vi "range_inc.vi"(8 "Error In":errorcluster, 10 "Unit":string, 11 "Amp":dbl) -> (0 "Error Out":errorcluster, 2 "Amp Base":dbl, 3 "Amp String":dbl)   [LabVIEW 2021, in "Signal.lvlib"]
doc: "This VI is used to check the range while incrementing or decrementing."
uses:
  Signal.lvlib
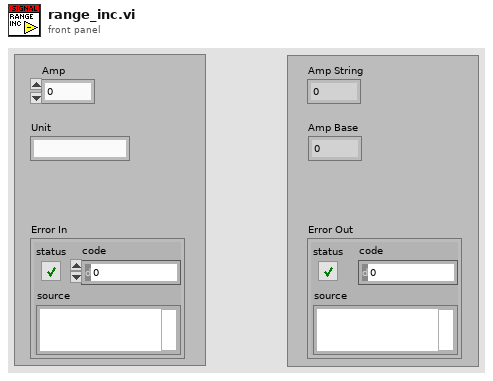
[diagram p1: front panel]
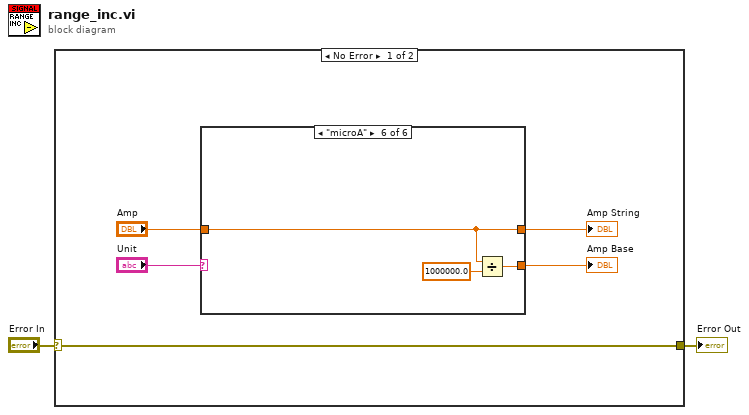
[diagram p0: block diagram]
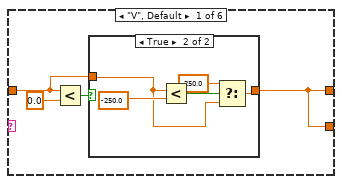
[diagram p2: hidden frame]
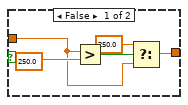
[diagram p3: hidden frame]
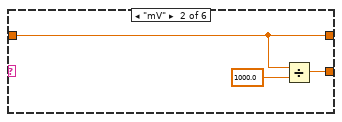
[diagram p4: hidden frame]
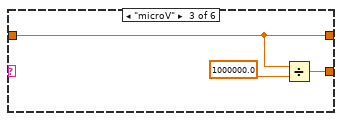
[diagram p5: hidden frame]
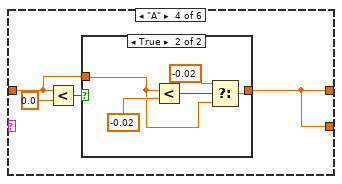
[diagram p6: hidden frame]
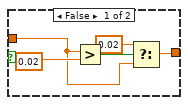
[diagram p7: hidden frame]
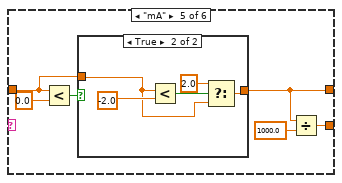
[diagram p8: hidden frame]
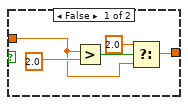
[diagram p9: hidden frame]
diagram:
  n1 = case shown="No Error" "Error In" {
    selector: "Error In" -> [w3 w61]
    tunnel: [w3 w61] -> w1
    frame No Error {
      n2 = case shown="\"microA\"" "Unit" {
        tunnel: "Amp" -> [w8 w23 w26 w29 w45 w59]
        tunnel: [w11 w22 w25 w28 w43 w60] -> w6
        tunnel: [w11 w23 w26 w28 w44 w59] -> w7
        frame "V", Default {
          n3 = Less?(x=w8, y=0.0) -> (x < y?=w9:bool)
          n4 = case shown="True" w9 {
            tunnel: [w13 w17] -> w11
            tunnel: w8 -> [w12 w18]
            frame False {
              n5 = Greater?(x=w12, y=250.0) -> (0:w15:bool)
              n6 = Select(t=250.0, s=w15, f=w12) -> (s? t:f=w13:dbl)
            }
            frame True {
              n7 = Less?(x=w18, y=-250.0) -> (x < y?=w20:bool)
              n8 = Select(t=-250.0, s=w20, f=w18) -> (s? t:f=w17:dbl)
            }
          }
        }
        frame "mV" {
          n9 = Divide(x=w23, y=1000.0) -> (x/y=w22:dbl)
        }
        frame "microV" {
          n10 = Divide(x=w26, y=1000000.0) -> (x/y=w25:dbl)
        }
        frame "A" {
          n11 = Less?(x=w29, y=0.0) -> (x < y?=w30:bool)
          n12 = case shown="True" w30 {
            tunnel: [w33 w37] -> w28
            tunnel: w29 -> [w32 w38]
            frame False {
              n13 = Greater?(x=w32, y=0.02) -> (0:w35:bool)
              n14 = Select(t=0.02, s=w35, f=w32) -> (s? t:f=w33:dbl)
            }
            frame True {
              n15 = Less?(x=w38, y=-0.02) -> (x < y?=w40:bool)
              n16 = Select(t=-0.02, s=w40, f=w38) -> (s? t:f=w37:dbl)
            }
          }
        }
        frame "mA" {
          n17 = Less?(x=w45, y=0.0) -> (x < y?=w46:bool)
          n18 = case shown="True" w46 {
            tunnel: [w49 w53] -> w44
            tunnel: w45 -> [w48 w54]
            frame False {
              n19 = Greater?(x=w48, y=2.0) -> (0:w51:bool)
              n20 = Select(t=2.0, s=w51, f=w48) -> (s? t:f=w49:dbl)
            }
            frame True {
              n21 = Less?(x=w54, y=-2.0) -> (x < y?=w56:bool)
              n22 = Select(t=2.0, s=w56, f=w54) -> (s? t:f=w53:dbl)
            }
          }
          n23 = Divide(x=w44, y=1000.0) -> (x/y=w43:dbl)
        }
        frame "microA" {
          n24 = Divide(x=w59, y=1000000.0) -> (x/y=w60:dbl)
        }
      }
      "Amp String" <- w7
      "Amp Base" <- w6
    }
    frame Error {
    }
  }
  "Error Out" <- w1
